vi "Concatenate String Array.vi"(4 "Max Number of Elements (None: -1)":i32=-1, 6 "Separator (TAB)":string="\t", 8 "Suffix (\"\")":string, 10 "String Array":string[](array[string]), 11 "Prefix (\"\")":string) -> (2 "Formatted String":string)   [LabVIEW 2021]
doc: "Concatenate a <B>String Array</B> into a single string, each element being separated by a <B>Separator</B> string (default: TAB), and the final string bracketed by the <B>Prefix</B> and <B>Suffix</B> strings.\n\nIf the array is empty, an empty string is returned.\n\nIf the array contains a single string, that string is returned.\n\nIf the user provides a <B>Max Number of Elements</B> parameter, the string array size is compared to it, and the output is limited to the first and last string, with an ellispsis in between."
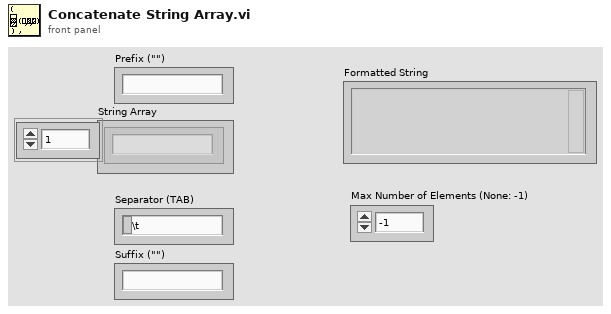
[diagram p1: front panel]
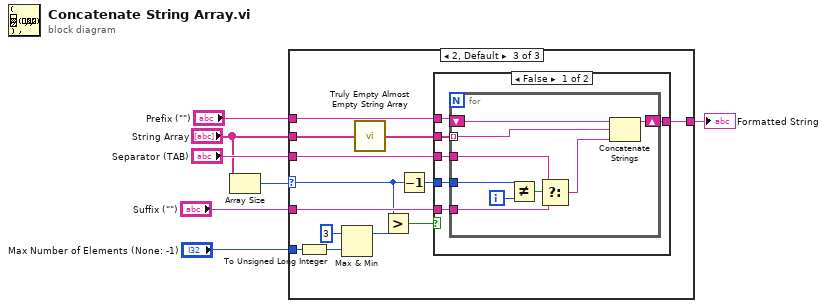
[diagram p0: block diagram]
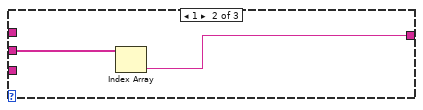
[diagram p3: hidden frame]
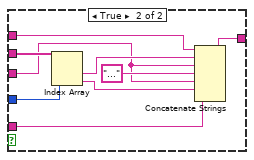
[diagram p4: hidden frame]
diagram:
  n1 = Array Size(array="String Array") -> (size(s)=w2:i32)
  n2 = case shown="2, Default" w2 {
    selector: w2 -> [_ _ w16]
    tunnel: [_ w8 w22] -> w7
    tunnel: "Prefix (\"\")" -> [_ _ w21]
    tunnel: "Separator (TAB)" -> [_ _ w20]
    tunnel: "String Array" -> [_ w9 w19]
    tunnel: "Suffix (\"\")" -> [_ _ w17]
    tunnel: "Max Number of Elements (None: -1)" -> [_ _ w15]
    frame 0 {
    }
    frame 1 {
      n3 = Index Array(array=w9) -> (element=w8:string)  [unwired: 1 in]
    }
    frame 2, Default {
      n4 = To Unsigned Long Integer(number=w15) -> (unsigned 32bit integer=w14:u32)
      n5 = Max & Min(x=u32 3, y=w14) -> (max(x,y)=w12:u32)  [unwired: 1 out]
      n6 = call "Truly Empty Almost Empty String Array.vi"("String Array"=w19) -> ("String Array"=w10:string[])  [unwired: 14 in]
      n7 = Greater?(x=w16, y=w12) -> (0:w13:bool)
      n8 = Decrement(x=w16) -> (x-1=w18:i32)
      n9 = case shown="False" w13 {
        tunnel: [w28 w38] -> w22
        tunnel: w21 -> [w27 w44]
        tunnel: w20 -> [w26 w40]
        tunnel: w10 -> [w25 w46]
        tunnel: w18 -> [w24 w45]
        tunnel: w17 -> [w23 w39]
        frame False {
          n10 = for {
            tunnel: w25 -> [w36] mode=indexing
            shift-right: [w35] -> w28
            shift-left: w27 -> [w37]
            tunnel: w26 -> [w30]
            tunnel: w24 -> [w34]
            tunnel: w23 -> [w31]
            i -> [w33]
            n11 = Not Equal?(x=w34, y=w33) -> (x != y?=w32:bool)
            n12 = Select(t=w30, s=w32, f=w31) -> (s? t:f=w29:string)
            n13 = Concatenate Strings(w37, w36, w29) -> (w35:string)
          }
        }
        frame True {
          n14 = Index Array(array=w46, index #2=w45) -> (element #1=w43:string, element #2=w41:string)  [unwired: 1 in]
          n15 = Concatenate Strings(w44, w43, w40, "..." ("string"), w40, w41, w39) -> (w38:string)
        }
      }
    }
  }
  "Formatted String" <- w7
